vi "updateScore.vi"(8 "error in":errorcluster, 11 "New Score":dbl) -> (0 "error out":errorcluster)   [LabVIEW 2024]
uses:
  session.vi
  <vilib>/httpClient/LabVIEWHTTPClient.lvlib
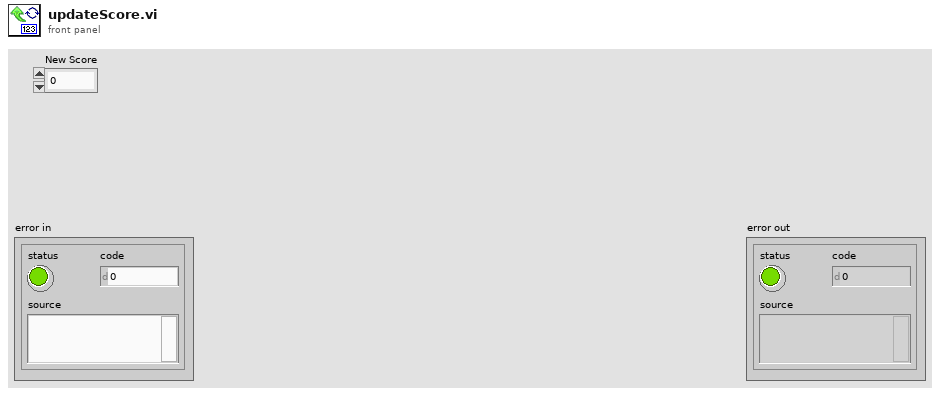
[diagram p1: front panel]
types:
  T1 = typedef "LabVIEWHTTPClient.lvlib/ClientHandle.ctl" = refnum<k1>
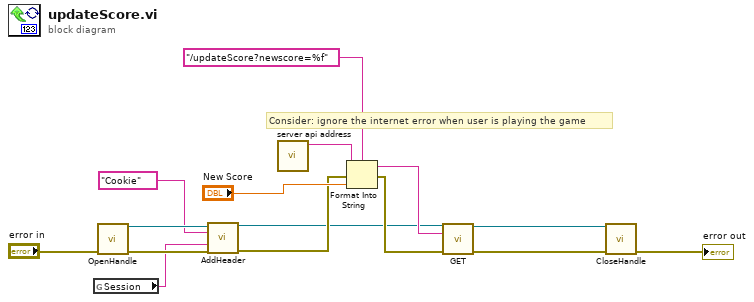
[diagram p0: block diagram]
diagram:
  # "Consider: ignore the internet error when user is playing the game"
  n1 = global read "session.vi" "Session"() -> (w1:string)
  n2 = call <vilib>:"OpenHandle.vi"("error in (no error)"="error in") -> ("client handle out"=w4:T1, "error out"=w6:errorcluster)  [unwired: 13 in]
  n3 = call <vilib>:"AddHeader.vi"("client handle"=w4, "header"="Cookie", "value"=w1, "error in (no error)"=w6) -> ("client handle out"=w3:T1, "error out"=w5:errorcluster)  [unwired: 10 in]
  n4 = call "server api address.vi"() -> ("Server API URL"=w10:string)  [unwired: 11 in]
  n5 = Format Into String(format string="/updateScore?newscore=%f", initial string=w10, error in=w5, "New Score") -> (resulting string=w7:string, error out=w8:errorcluster)
  n6 = call <vilib>:"GET.vi"("client handle"=w3, "url"=w7, "error in (no error)"=w8) -> ("client handle out"=w12:T1, "error out"=w13:errorcluster)  [unwired: 9 in, 2 out]
  n7 = call <vilib>:"CloseHandle.vi"("client handle"=w12, "error in (no error)"=w13) -> ("error out"=→"error out":errorcluster)  [unwired: 13 in]
